vi "WriteI2C.vi"(8 "error in (no error)":errorcluster, 9 "Write Data(Hex)":string="11 22 33 44 55 66 77 88", 10 "Reg Addr(Hex)":u8 format="%x", 11 "Slave Addr(Hex)":i16=80 format="%x") -> (0 "error out":errorcluster)   [LabVIEW 2024]
panel:
  in  "appended array":u8[](array[numeric]) format="%.0x"
  in  "接口电压":i8(ring)=3 items=["0 V", "1.8 V", "2.5 V", "3.3 V"]
  in  "Channel Index":i32(ring) items=["CH0", "CH1", "CH2", "CH3", "CH4", "CH5", "CH6", "CH7"]
  in  "pConfig":T1={"ClockSpeedHz"=100000, "OwnAddr"=0, "Master"=1, "AddrBits"=7, "EnablePu"=1, "ByteIntervalUs"=0}
  in  "Device Index":i32(ring) items=["0", "1", "2", "3", "4", "5"]
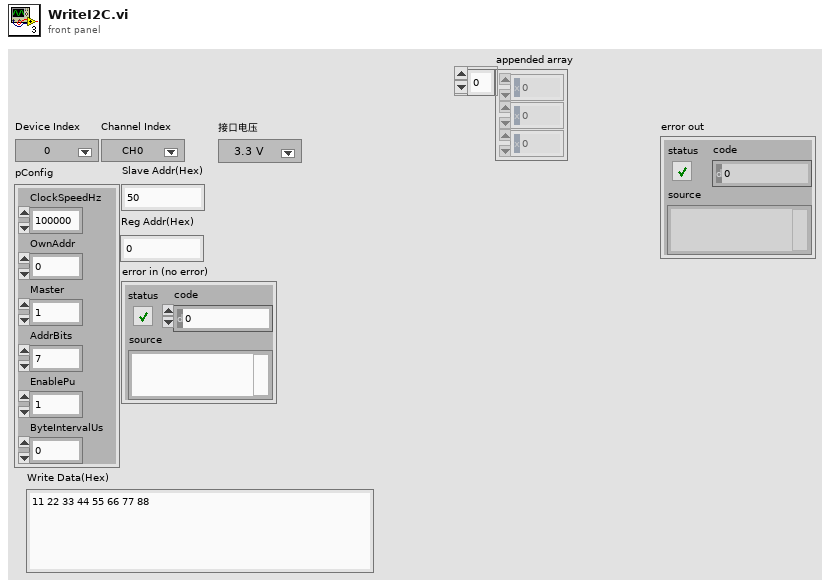
[diagram p1: front panel]
types:
  T1 = cluster{"ClockSpeedHz":u32, "OwnAddr":u16, "Master":u8, "AddrBits":u8, "EnablePu":u8, "ByteIntervalUs":u8}
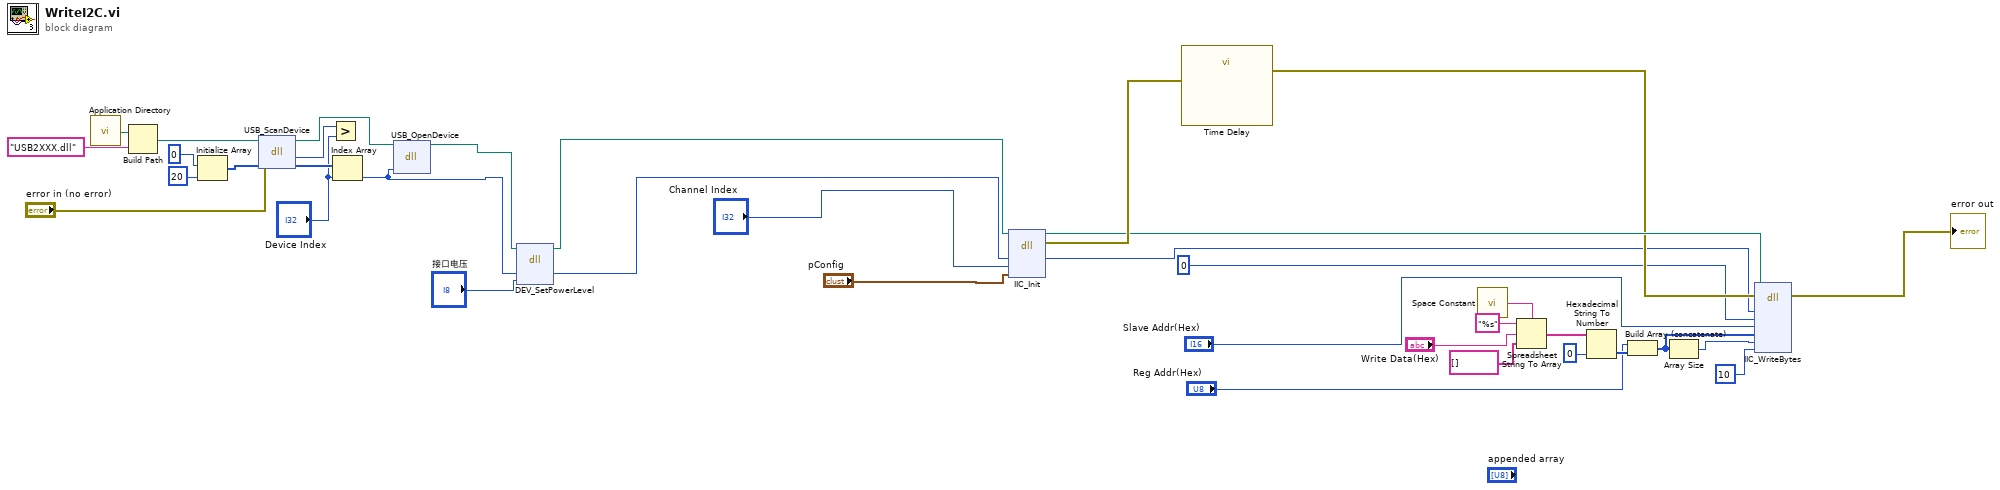
[diagram p0: block diagram]
diagram:
  n1 = call <vilib>:"Application Directory.vi"() -> ("Application Directory"=w30:path)
  n2 = Build Path(base path=w30, name or relative path="USB2XXX.dll") -> (appended path=w29:path)
  n3 = Initialize Array(0, 20 ("dimension size")) -> (w33:i32[])
  n4 = dll-call lib="D:/Project/Teststand/RFP Auto Test Sequence/Support/IIC/USB2XXX.dll" fn="USB_ScanDevice"(path in=w29, error in="error in (no error)", "pDevNum"=w33) -> (path out=w25:path, "return type"=w32:i32, "pDevNum"=w36:i32[])  [unwired: 1 in, 1 out]
  n5 = Greater?(x=w32, y="Device Index") -> ()  [unwired: 1 out]
  n6 = Index Array(array=w36, index="Device Index") -> (element=w23:i32)
  n7 = dll-call lib="D:/Project/Teststand/RFP Auto Test Sequence/Support/IIC/USB2XXX.dll" fn="USB_OpenDevice"(path in=w25, "DevIndex"=w23) -> (path out=w24:path)  [unwired: 4 in, 1 out]
  n8 = dll-call lib="D:/Project/Teststand/RFP Auto Test Sequence/Support/IIC/USB2XXX.dll" fn="DEV_SetPowerLevel"(path in=w24, "DevHandle"=w23, "PowerLevel"="接口电压") -> (path out=w22:path, "DevHandle"=w20:i32)  [unwired: 4 in, 1 out]
  n9 = dll-call lib="D:/Project/Teststand/RFP Auto Test Sequence/Support/IIC/USB2XXX.dll" fn="IIC_Init"(path in=w22, "DevIndex"=w20, "IICIndex"="Channel Index", "pConfig"="pConfig") -> (path out=w7:path, error out=w19:errorcluster, "DevIndex"=w1:i32)  [unwired: 5 in]
  n10 = call "Time Delay"("error in (no error)"=w19) -> ("error out"=w6:errorcluster)  [unwired: 10 in]
  n11 = call <vilib>:"Space Constant.vi"() -> ("String"=w13:string)
  n12 = Spreadsheet String To Array(delimiter (Tab)=w13, format string="%s", spreadsheet string="Write Data(Hex)", array type (2D Dbl)=string[] []) -> (array=w16:string[])
  n13 = Hexadecimal String To Number(string=w16, default (0uL)=u8 0 ("default (0 U32)")) -> (number=w10:u8[])  [unwired: 1 in, 1 out]
  n14 = Build Array (concatenate)("Reg Addr(Hex)", w10) -> (w2:u8[])
  n15 = Array Size(array=w2) -> (size(s)=w9:i32)
  n16 = dll-call lib="D:/Project/Teststand/RFP Auto Test Sequence/Support/IIC/USB2XXX.dll" fn="IIC_WriteBytes"(path in=w7, error in=w6, "DevIndex"=w1, "IICIndex"=0, "SlaveAddr"="Slave Addr(Hex)", "pWriteData"=w2, "WriteLen"=w9, "TimeOutMs"=10) -> (error out=→"error out":errorcluster)  [unwired: 8 in, 1 out]
